vi "GetTextPositions.vi"(0 "reference":refnum<class "SegmentedLineEdge.lvclass">, 1 "GraphicsRef":refnum<class "Graphics.lvclass">, 5 "error in (no error)":errorcluster) -> (14 "reference out":refnum<class "SegmentedLineEdge.lvclass">, 15 "connectionPoints":T1[](array[typedef]) {"y" format="%.2f"; "x" format="%.2f"}, 19 "error out":errorcluster)   [LabVIEW 2014, in "SegmentedLineEdge.lvclass"]
doc: "GetTextPositions"
uses:
  <resource>/Framework/Providers/Open_GDS/UML/SegmentedLineEdge_class/SegmentedLineEdge.lvclass
  <resource>/Framework/Providers/Open_GDS/UML/General/Point/Point Point2D.ctl
  <resource>/Framework/Providers/Open_GDS/UML/Graphics_class/Graphics.lvclass
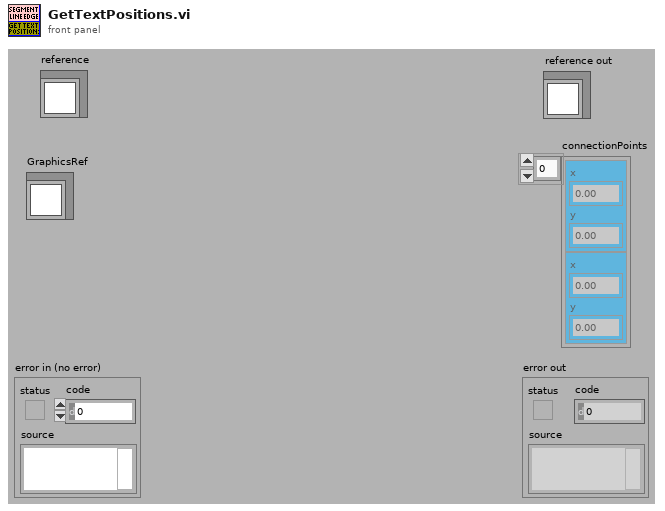
[diagram p1: front panel]
types:
  T1 = typedef "Point Point2D.ctl" = cluster{"x":dbl, "y":dbl}
  T2 = typedef "SegmentedLineEdge.lvclass/ObjectAttributes.ctl" = cluster{"lineStyle":refnum<class "LineStyle.lvclass">, "startArrowHead":refnum<class "ArrowHead.lvclass">, "endArrowHead":refnum<class "ArrowHead.lvclass">, "startLabel":string, "midLabel":string, "endLabel":string, "MidLabelOffset":T1, "SplitWire":bool}
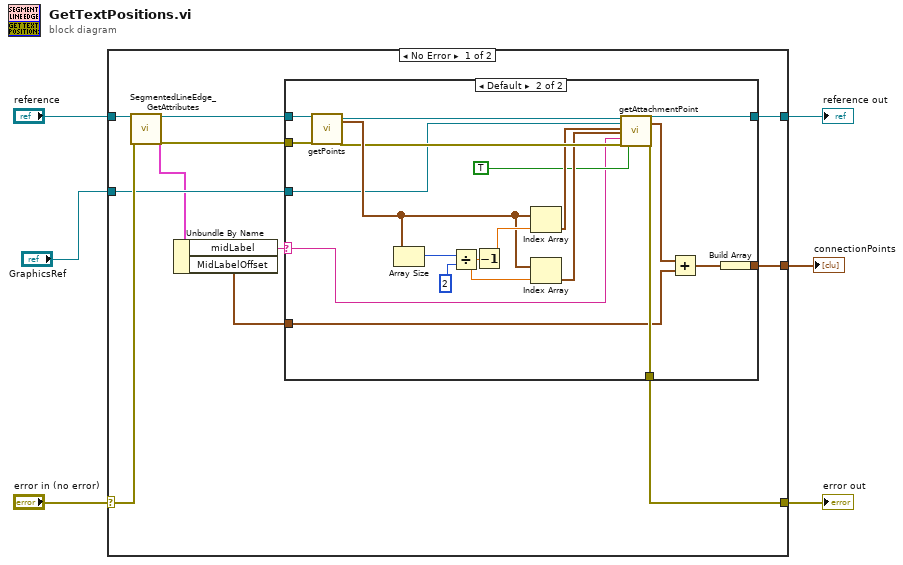
[diagram p0: block diagram]
diagram:
  n1 = case shown="No Error" "error in (no error)" {
    selector: "error in (no error)" -> [w17 w40]
    tunnel: "reference" -> [w16 w41]
    tunnel: [w11 w40] -> w4
    tunnel: [w13 w41] -> w3
    tunnel: [w12 _] -> w2
    tunnel: "GraphicsRef" -> [w8 _]
    frame No Error {
      n2 = call <resource>:"SegmentedLineEdge_GetAttributes.vi"("reference in"=w16, "error in (no error)"=w17) -> ("reference out"=w14:refnum<class "SegmentedLineEdge.lvclass">, "Data"=w7:T2, "error out"=w15:errorcluster)  [unwired: 1 in, 14 out]
      n3 = Unbundle By Name(w7) -> ("midLabel"=w10:string, "MidLabelOffset"=w9:T1)
      n4 = case shown="Default" w10 {
        selector: w10 -> [_ w20]
        tunnel: w15 -> [w18 w34]
        tunnel: w14 -> [w19 w33]
        tunnel: [w19 w32] -> w13
        tunnel: [_ w28] -> w12
        tunnel: [w18 w27] -> w11
        tunnel: w9 -> [_ w22]
        tunnel: w8 -> [_ w21]
        frame "" {
        }
        frame Default {
          n5 = call-dynamic "getPoints.vi"("reference"=w33, "error in (no error)"=w34) -> ("reference out"=w25:refnum<class "SegmentedLineEdge.lvclass">, "points"=w36:T1[], "error out"=w31:errorcluster)  [unwired: 15 in]
          n6 = Array Size(array=w36) -> (size(s)=w39:i32)
          n7 = Divide(x=w39, y=2) -> (x/y=w35:dbl)
          n8 = Decrement(x=w35) -> (x-1=w37:dbl)
          n9 = Index Array(array=w36, index=w37) -> (element=w30:T1)
          n10 = Index Array(array=w36, index=w35) -> (element=w29:T1)
          n11 = call-dynamic "getAttachmentPoint.vi"("reference"=w25, "graphics"=w21, "p1"=w30, "p2"=w29, "text"=w20, "error in (no error)"=w31, "center"=TRUE) -> ("reference out"=w32:refnum<class "SegmentedLineEdge.lvclass">, "attachPoint"=w23:T1, "error out"=w27:errorcluster)  [unwired: 10 in]
          n12 = Add(x=w23, y=w22) -> (x+y=w24:T1)
          n13 = Build Array(w24) -> (w28:T1[])
        }
      }
    }
    frame Error {
    }
  }
  "reference out" <- w3
  "error out" <- w4
  "connectionPoints" <- w2
